vi "set_channel_number.vi"(8 "error in (no error)":errorcluster, 10 "file name":string, 11 "TrajectoryMH100122AODRAPS in":refnum<class "TrajectoryMH100122AODRAPS.lvclass">) -> (0 "error out":errorcluster, 3 "TrajectoryMH100122AODRAPS out":refnum<class "TrajectoryMH100122AODRAPS.lvclass">)   [LabVIEW 2010, in "TrajectoryMH100122AODRAPS.lvclass"]
uses:
  TrajectoryMH100122AODRAPS.lvclass
  TrajectoryMH100122AODRAPS.lvclass/TrajectoryMH100122AODRAPS.ctl
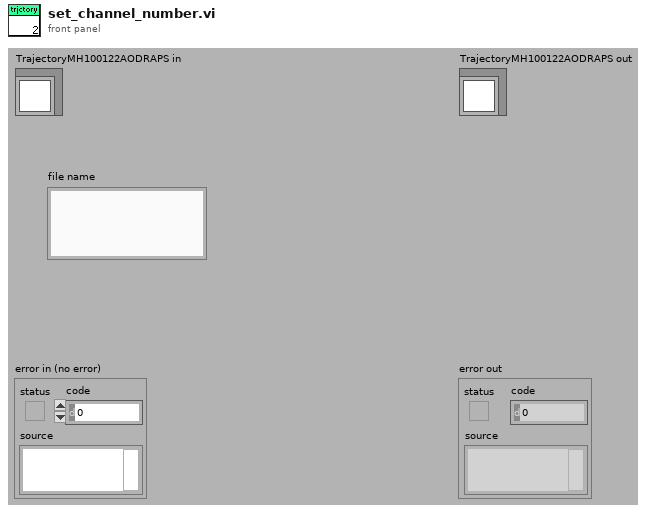
[diagram p1: front panel]
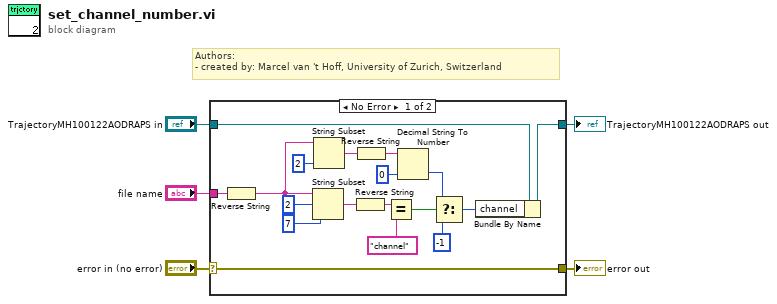
[diagram p0: block diagram]
diagram:
  # "Authors: \n- created by: Marcel van 't Hoff, University of Zurich, Switzerland"
  n1 = case shown="No Error" "error in (no error)" {
    selector: "error in (no error)" -> [w23 w25]
    tunnel: [w23 w25] -> w4
    tunnel: [w8 w24] -> w2
    tunnel: "TrajectoryMH100122AODRAPS in" -> [w9 w24]
    tunnel: "file name" -> [w22 _]
    frame No Error {
      n2 = Reverse String(1:w22) -> (0:w16:string)
      n3 = String Subset(string=w16, offset (0)=2, length (rest)=7 ("length (rest)")) -> (substring=w20:string)
      n4 = String Subset(string=w16, length (rest)=2 ("length (rest)")) -> (substring=w14:string)  [unwired: 1 in]
      n5 = Reverse String(1:w20) -> (0:w18:string)
      n6 = Reverse String(1:w14) -> (0:w13:string)
      n7 = Equal?(x=w18, y="channel") -> (x = y?=w12:bool)
      n8 = Decimal String To Number(string=w13, default (0L)=i8 0 ("default (0 I32)")) -> (number=w11:i8)  [unwired: 1 in, 1 out]
      n9 = Select(t=w11, s=w12, f=i8 -1) -> (s? t:f=w7:i8)
      n10 = Bundle By Name(cluster=w9, "channel"=w7) -> (w8:refnum<class "TrajectoryMH100122AODRAPS.lvclass">)
    }
    frame Error {
    }
  }
  "error out" <- w4
  "TrajectoryMH100122AODRAPS out" <- w2
